vi "HTTP_Write.vi"(6 "Server":path, 8 "error in (no error)":errorcluster, 11 "Code":string) -> (0 "error out":errorcluster)   [LabVIEW 2020]
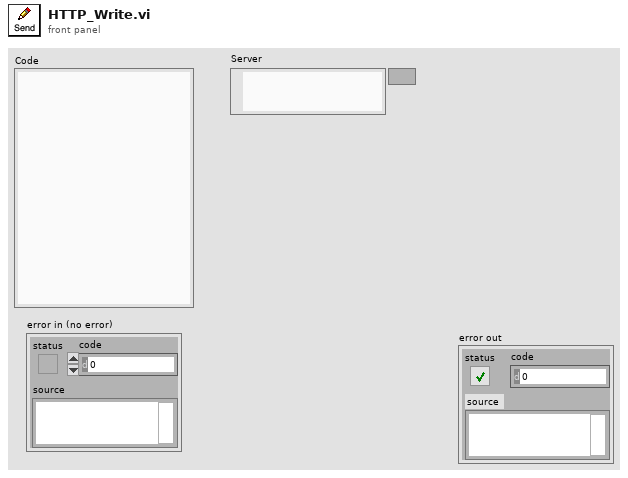
[diagram p1: front panel]
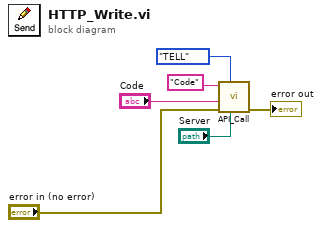
[diagram p0: block diagram]
diagram:
  n1 = call "API_Call.vi"("Server"="Server", "Direction"=enum16{"ASK", "TELL"}."TELL", "error in (no error)"="error in (no error)", "Payload"="Code", "cmd"="Code" ("url")) -> ("error out"=→"error out":errorcluster)  [unwired: 3 in, 3 out]
